vi "Center UI over Caller.vi"(8 "error in":errorcluster, 10 "Calling VI":refnum<vi>, 11 "VI to Center":refnum<vi>) -> (0 "error out":errorcluster)   [LabVIEW 2014, in "Flex UI Dialog.lvclass"]
doc: "Centers the input VI on the specified Calling VI."
uses:
  Flex UI Dialog.lvclass
  <vilib>/XNodeSupport/NI_XNodeSupport.lvlib
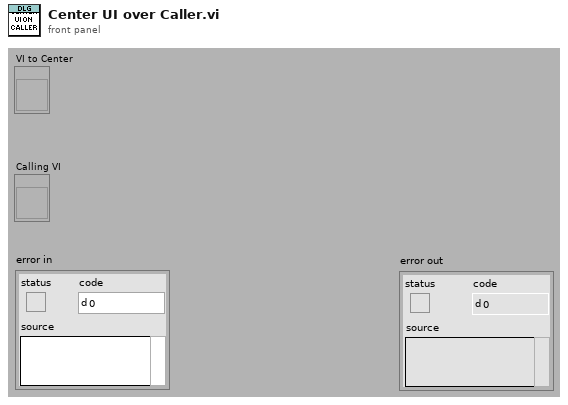
[diagram p1: front panel]
types:
  T1 = typedef "LVRectTypeDef.ctl" = cluster{"Left":i16, "Top":i16, "Right":i16, "Bottom":i16}
  T2 = typedef "NI_XNodeSupport.lvlib/XNodeBounds.ctl" = cluster{"Width":T3, "Height":T3}
  T3 = typedef "NI_XNodeSupport.lvlib/XNodeInt.ctl" = i32
  T4 = typedef "NI_XNodeSupport.lvlib/XNodeRect32.ctl" = cluster{"Left":T3, "Top":T3, "Right":T3, "Bottom":T3}
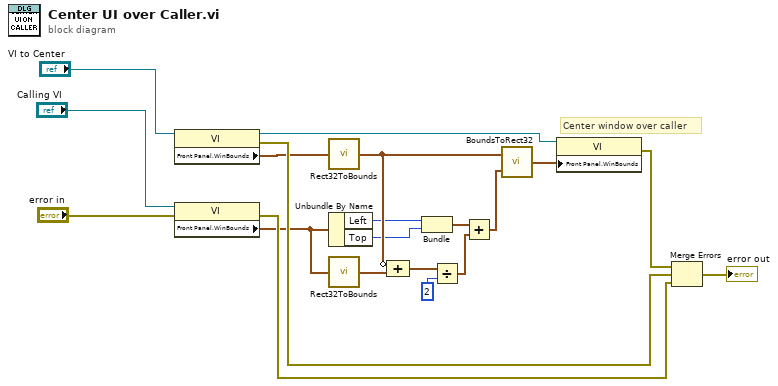
[diagram p0: block diagram]
diagram:
  # "Center window over caller"
  n1 = property class="VI"(reference="VI to Center") -> (reference out=w17:refnum<vi>, error out=w19:errorcluster, "Front Panel.WinBounds"=w16:T1)  [unwired: 1 in]
  n2 = property class="VI"(reference="Calling VI", error in="error in") -> (error out=w20:errorcluster, "Front Panel.WinBounds"=w12:T1)  [unwired: 1 out]
  n3 = call <vilib>:"Rect32ToBounds.vi"("Rect32"=w16) -> ("Bounds"=w18:T2)
  n4 = Unbundle By Name(w12) -> ("Left"=w10:i16, "Top"=w11:i16)
  n5 = call <vilib>:"Rect32ToBounds.vi"("Rect32"=w12) -> ("Bounds"=w6:T2)
  n6 = Compound Arithmetic op=ADD(invert w18, w6) -> (w14:T2)
  n7 = Bundle("Left"=w10, "Top"=w11) -> (w8:cluster{"Left":i16, "Top":i16})  [unwired: 1 out]
  n8 = Divide(x=w14, y=2) -> (x/y=w9:cluster{"Width":dbl, "Height":dbl})
  n9 = Add(x=w8, y=w9) -> (x+y=w7:cluster{dbl, dbl})
  n10 = call <vilib>:"BoundsToRect32.vi"("Offset (0,0)"=w7, "Bounds"=w18) -> ("Rect32"=w15:T4)
  n11 = property class="VI"(reference=w17, "Front Panel.WinBounds"=w15) -> (error out=w1:errorcluster)  [unwired: 1 in, 1 out]
  n12 = Merge Errors(w1, w19, w20) -> (→"error out":errorcluster)
